vi "ConvertLEDMessage.vi"(11 "ROS Info":T1={"Node Name"="Node", "Topic Name"="/cmd_lightring", "Message Type"="irobot_create_msgs/msg/LightringLeds", "Message"="{\"override_system\":true,\"leds\":[{\"red\":255,\"green\":0,\"blue\":0},{\"red\":4,\"green\":255,\"blue\":0},{\"red\":6,\"green\":0,\"blue\":255},{\"red\":239,\"green\":142,\"blue\":0},{\"red\":226,\"green\":0,\"blue\":255},{\"red\":0,\"green\":250,\"blue\":255}]}", "Pub_Time"="5"}) -> (3 "ROS corrected":T1={"Node Name"="Node", "Topic Name"="/cmd_lightring", "Message Type"="irobot_create_msgs/msg/LightringLeds", "Message"="{\"override_system\":true,\"leds\":[{\"red\":255,\"green\":0,\"blue\":0},{\"red\":4,\"green\":255,\"blue\":0},{\"red\":6,\"green\":0,\"blue\":255},{\"red\":239,\"green\":142,\"blue\":0},{\"red\":226,\"green\":0,\"blue\":255},{\"red\":0,\"green\":250,\"blue\":255}]}", "Pub_Time"="5"})   [LabVIEW 2022 SP3]
uses:
  ROSCtrl.ctl
panel:
  # "-1 means \nsubscribe"
  # "-1 means \nsubscribe"
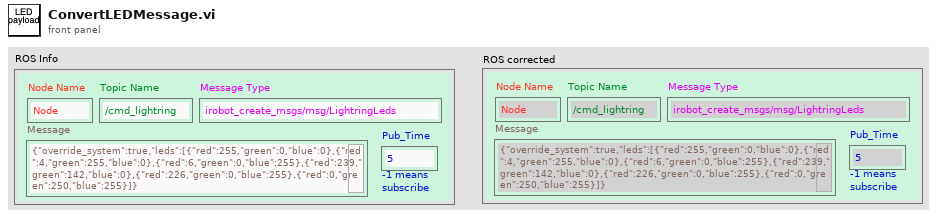
[diagram p1: front panel]
types:
  T1 = typedef "ROSCtrl.ctl" = cluster{"Node Name":string, "Topic Name":string, "Message Type":string, "Message":string, "Pub_Time":string}
  T2 = cluster{"override_system":bool, "leds":cluster{"red":u8, "green":u8, "blue":u8}[]}
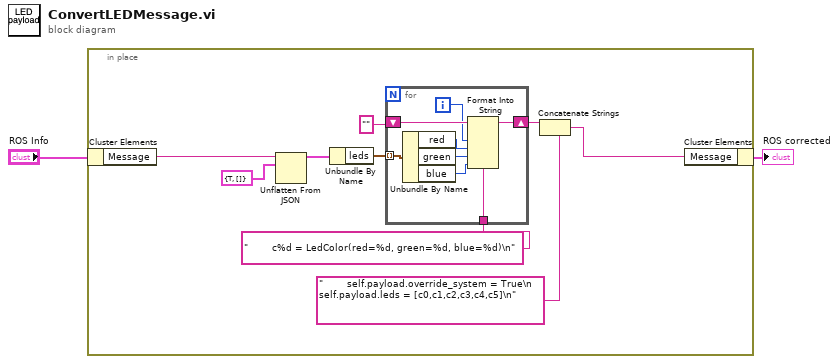
[diagram p0: block diagram]
diagram:
  n1 = in-place {
    n2 = in-place-cluster #1("ROS Info") -> ("Message"=w4:string)
    n3 = Unflatten From JSON(JSON string=w4, type and defaults=T2 {"override_system"=TRUE, "leds"=[]}) -> (value=w11:T2)  [unwired: 5 in, 1 out]
    n4 = Unbundle By Name(w11) -> ("leds"=w10:cluster{"red":u8, "green":u8, "blue":u8}[])
    n5 = for {
      tunnel: w10 -> [w19] mode=indexing
      tunnel: "        c%d = LedColor(red=%d, green=%d, blue=%d)\n" ("search string") -> [w18]
      shift-right: [w13] -> w9
      shift-left: "" ("search string") -> [w14]
      i -> [w12]
      n6 = Unbundle By Name(w19) -> ("red"=w17:u8, "green"=w15:u8, "blue"=w16:u8)
      n7 = Format Into String(format string=w18, initial string=w14, w12, w17, w15, w16) -> (resulting string=w13:string)  [unwired: 1 in, 1 out]
    }
    n8 = Concatenate Strings(w9, "        self.payload.override_system = True\n        self.payload.leds = [c0,c1,c2,c3,c4,c5]\n" ("search string")) -> (w3:string)
    n9 = in-place-cluster #1("Message"=w3) -> (→"ROS corrected":T1)
  }
